vi "niRFUtil FTW Generate Gaussian FIR Filter.vi"(1 "Minimum Selectivity (dB)":dbl=70.0 format="%.2f", 2 "Sampling Rate (Hz)":dbl=2160000.0 format="%^.3e", 3 "Bandwidth (Hz)":dbl=300000.0 format="%^.3e") -> (0 "Filter":T1={"x0"=-2.777777777777778e-06, "dx"=4.6296296296296297e-07, "y"=[]} {"y" min=0 max=127 format="%.2f"; "dx" format="%^.2e"; "x0" format="%^.2e"})   [LabVIEW 2016, in "niRFUtil.lvlib"]
doc: "(c) Copyright 2006, National Instruments, Inc. This VI may not be duplicated, sold, or distributed without written consent from National Instruments."
uses:
  niRFUtil.lvlib
  Includes/niRFUtil INC Real Waveform.ctl
  Includes/niRFUtil INC Real Array.ctl
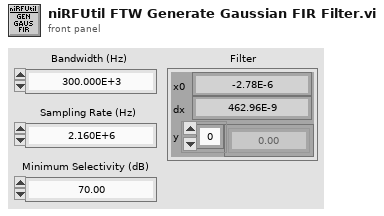
[diagram p1: front panel]
types:
  T1 = typedef "niRFUtil.lvlib/niRFUtil INC Real Waveform.ctl" = cluster{"x0":dbl, "dx":dbl, "y":T2}
  T2 = typedef "niRFUtil.lvlib/niRFUtil INC Real Array.ctl" = sgl[]
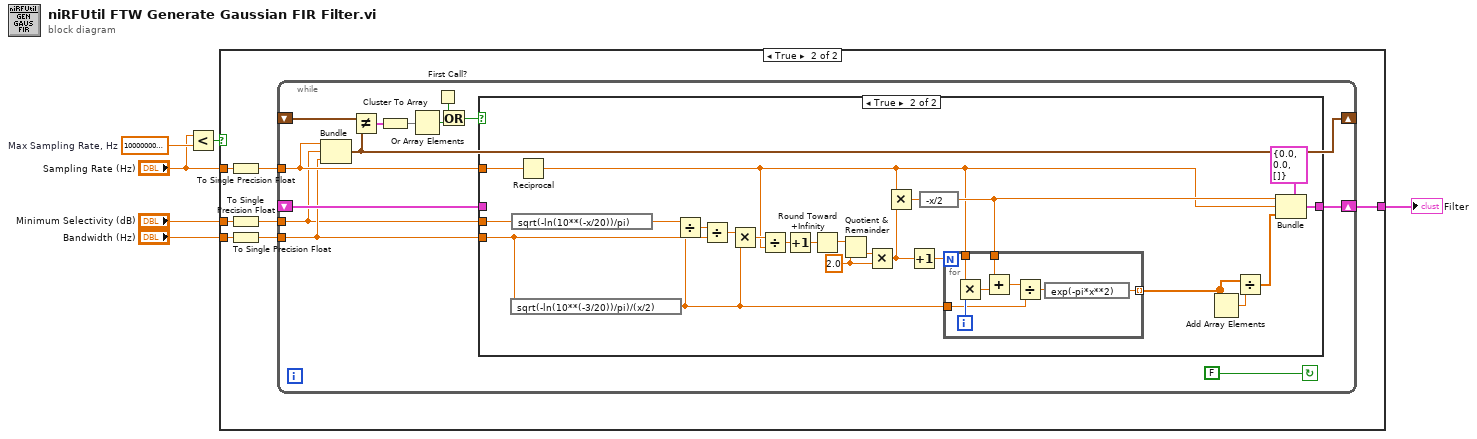
[diagram p0: block diagram]
diagram:
  w3 = 1000000000.0  # Max Sampling Rate, Hz
  n1 = Less?(x="Sampling Rate (Hz)", y=w3) -> (x < y?=w1:bool)
  n2 = case shown="True" w1 {
    tunnel: "Bandwidth (Hz)" -> [_ w13]
    tunnel: "Sampling Rate (Hz)" -> [_ w12]
    tunnel: [_ w11] -> w5
    tunnel: "Minimum Selectivity (dB)" -> [_ w10]
    frame False {
    }
    frame True {
      n3 = To Single Precision Float(number=w12) -> (single precision float=w9:sgl)
      n4 = To Single Precision Float(number=w10) -> (single precision float=w8:sgl)
      n5 = To Single Precision Float(number=w13) -> (single precision float=w7:sgl)
      n6 = while {
        shift-right: [w25] -> w11
        shift-left: _ -> [w24]
        tunnel: w9 -> [w18]
        tunnel: w7 -> [w15]
        shift-right: [w16] -> _
        shift-left: _ -> [w17]
        tunnel: w8 -> [w14]
        stop <- FALSE continue-if-true
        n7 = Bundle(w18, w14, w15) -> (w16:cluster{sgl, sgl, sgl})  [unwired: 1 out]
        n8 = Not Equal?(x=w17, y=w16) -> (x != y?=w19:cluster{bool, bool, bool})
        n9 = Cluster To Array(cluster=w19) -> (array=w23:bool[])
        n10 = Or Array Elements(Boolean array=w23) -> (logical OR=w22:bool)
        n11 = First Call?() -> (First Call?: T/F=w21:bool)
        n12 = Or(x=w21, y=w22) -> (x .or. y?=w20:bool)
        n13 = case shown="True" w20 {
          tunnel: [w27 w49] -> w25
          tunnel: w24 -> [w27 _]
          tunnel: w18 -> [_ w46]
          tunnel: w15 -> [_ w36]
          tunnel: w14 -> [_ w47]
          frame False {
          }
          frame True {
            w42 = sgl 2.0 ("y")
            n14 = expression code="sqrt(-ln(10**(-3/20))/pi)/(x/2)"(w36) -> (w34:sgl)
            n15 = expression code="sqrt(-ln(10**(-x/20))/pi)"(w47) -> (w48:sgl)
            n16 = Reciprocal(x=w46) -> (1/x=w32:sgl)
            n17 = Divide(x=w48, y=w34) -> (x/y=w45:sgl)
            n18 = Divide(x=w45, y=w36) -> (x/y=w35:sgl)
            n19 = Multiply(x=w35, y=w34) -> (x*y=w33:sgl)
            n20 = Divide(x=w33, y=w32) -> (x/y=w29:sgl)
            n21 = Increment(x=w29) -> (x+1=w41:sgl)
            n22 = Round Toward +Infinity(x=w41) -> (ceil(x): smallest int >= x=w44:sgl)
            n23 = Quotient & Remainder(x=w44, y=w42) -> (floor(x/y)=w43:sgl)  [unwired: 1 out]
            n24 = Multiply(x=w43, y=w42) -> (x*y=w40:sgl)
            n25 = Multiply(x=w32, y=w40) -> (x*y=w39:sgl)
            n26 = Increment(x=w40) -> (x+1=w37:sgl)
            n27 = expression code="-x/2"(w39) -> (w38:sgl)
            n28 = for {
              N: w37 -> [_]
              tunnel: w34 -> [w55]
              tunnel: [w53] -> w30 mode=indexing
              tunnel: w32 -> [w52]
              tunnel: w38 -> [w51]
              i -> [w58]
              n29 = Multiply(x=w52, y=w58) -> (x*y=w57:sgl)
              n30 = Add(x=w51, y=w57) -> (x+y=w56:sgl)
              n31 = Divide(x=w56, y=w55) -> (x/y=w54:sgl)
              n32 = expression code="exp(-pi*x**2)"(w54) -> (w53:sgl)
            }
            n33 = Add Array Elements(numeric array=w30) -> (sum=w50:sgl)
            n34 = Divide(x=w30, y=w50) -> (x/y=w31:sgl[])
            n35 = Bundle(cluster=T1 {"x0"=0.0, "dx"=0.0, "y"=[]} ("Filter"), "x0"=w38, "dx"=w32, "y"=w31) -> (w49:T1)
          }
        }
      }
    }
  }
  "Filter" <- w5
